vi "usrp get tx antennas.vi"(8 "error in (no error)":errorcluster, 9 "antennas_out":u64, 10 "chan":u64, 11 "h":u64) -> (0 "error out":errorcluster, 1 "antennas_out out":u64, 2 "function return":u32(ring), 3 "h 2":u64)   [LabVIEW 2024, in "uhd.lvlib"]
doc: "UHD_API uhd_error uhd_usrp_get_tx_antennas(\n uhd_usrp_handle h, size_t chan, uhd_string_vector_handle* antennas_out);"
uses:
  uhd.lvlib
  uhd.so
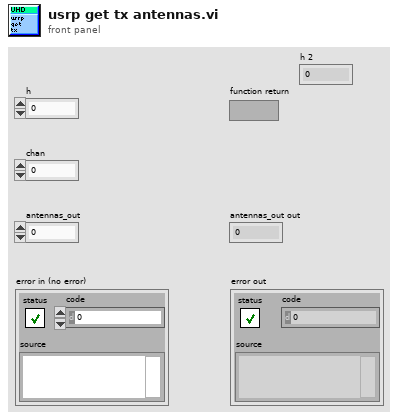
[diagram p1: front panel]
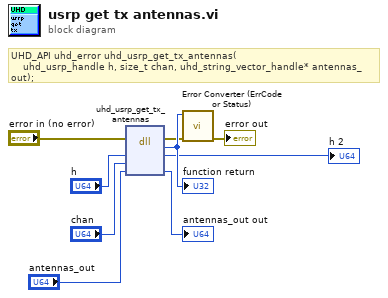
[diagram p0: block diagram]
diagram:
  # "UHD_API uhd_error uhd_usrp_get_tx_antennas(\n    uhd_usrp_handle h, size_t chan, uhd_string_vector_handle* antennas_out);"
  n1 = dll-call lib="uhd.*" fn="uhd_usrp_get_tx_antennas"(error in="error in (no error)", "h"="h", "chan"="chan", "antennas_out"="antennas_out") -> (error out=w3:errorcluster, w9:u32, "h"=→"h 2":u64, "antennas_out"=→"antennas_out out":u64)  [unwired: 3 in, 1 out]
  "function return" <- w9
  n2 = call "Error Converter (ErrCode or Status).vi"("error in (no error)"=w3, "error code"=w9) -> ("error out"=→"error out":errorcluster)  [unwired: 9 in]
